vi "Group.Create.vi"(8 "error in (no error)":errorcluster, 9 "Name":string, 11 "Parent":T1 format="%.0x") -> (0 "error out":errorcluster, 2 "Child":T1 format="%.0x", 3 "Parent":T1 format="%.0x")   [LabVIEW 2019, in "Fuel Injector Analysis Addon System Explorer.lvlib"]
uses:
  Fuel Injector Analysis Addon System Explorer.lvlib
  <vilib>/NI VeriStand/Custom Device API/Custom Device Item Ref.ctl
  Addon Shared/Constants.vi
  <vilib>/NI VeriStand/Custom Device Tools/Custom Device Utility Library/NI VeriStand - Search for All Items by GUID.vi
  <vilib>/NI VeriStand/Custom Device Tools/Custom Device Utility Library/Custom Device Utility Library.lvlib
  <vilib>/NI VeriStand/Custom Device API/Custom Device API.lvlib
  Addon Shared/Fuel Injector Analysis Addon Shared.lvlib
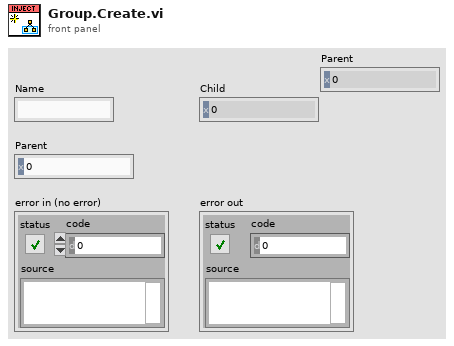
[diagram p1: front panel]
types:
  T1 = typedef "Custom Device API.lvlib/Custom Device Item Ref.ctl" = u64
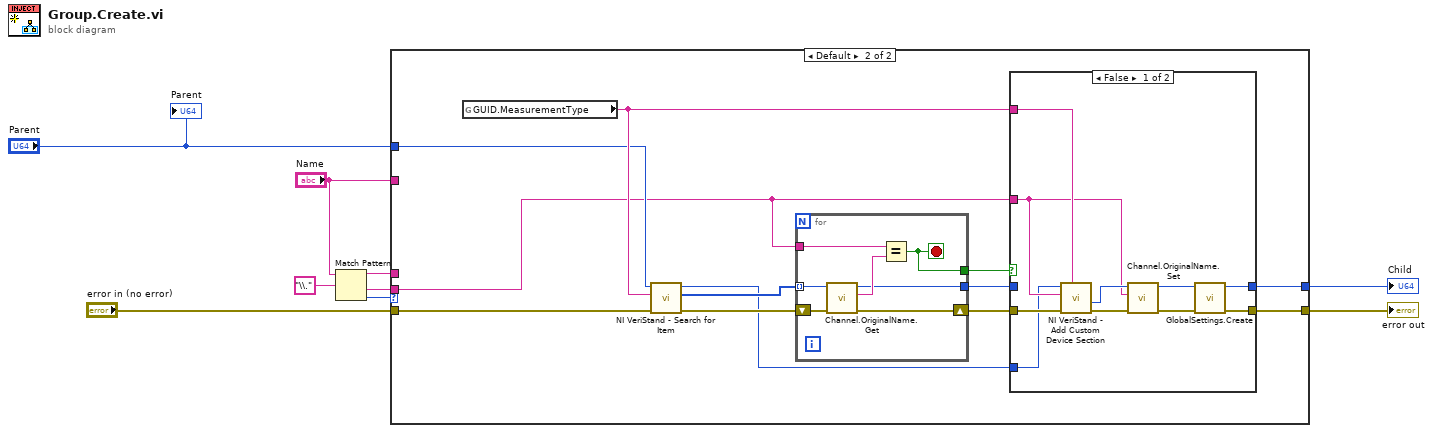
[diagram p0: block diagram]
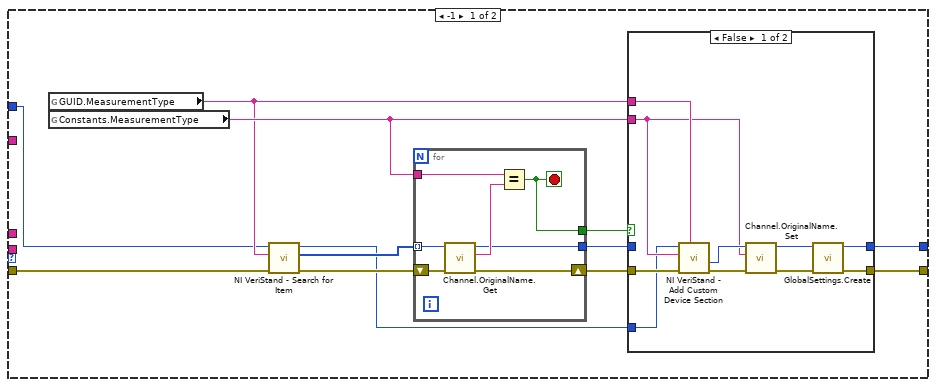
[diagram p2: hidden frame]
diagram:
  n1 = Match Pattern(string="Name", regular expression="\\.") -> (before substring=w4:string, after substring=w9:string, offset past match=w2:i32)  [unwired: 1 in, 1 out]
  n2 = case shown="Default" w2 {
    tunnel: "error in (no error)" -> [w10 w42]
    tunnel: w4 -> [_ _]
    tunnel: "Parent" -> [w11 w43]
    tunnel: [w21 w52] -> w5
    tunnel: [w20 w51] -> w7
    tunnel: "Name" -> [_ _]
    tunnel: w9 -> [_ w41]
    frame -1 {
      n3 = global read "Constants.vi" "GUID.MeasurementType"() -> (w12:string)
      n4 = global read "Constants.vi" "Constants.MeasurementType"() -> (w13:string)
      n5 = call-poly <vilib>:"NI VeriStand - Search for Item.vi"("error in"=w10, "Item GUID"=w12, "Section Ref in"=w11) -> ("error out"=w19:errorcluster, "Item Refs"=w18:T1[], "Section Ref out"=w14:T1)  [unwired: 5 in, 1 out]
      n6 = for {
        shift-right: [w27] -> w17
        shift-left: w19 -> [w28]
        tunnel: w18 -> [w26] mode=indexing
        tunnel: w13 -> [w24]
        tunnel: [w23] -> w15
        tunnel: [w22] -> w16
        stop <- w22 stop-if-true
        n7 = call "Channel.OriginalName.Get.vi"("error in (no error)"=w28, "Ref in"=w26) -> ("error out"=w27:errorcluster, "Value"=w25:string, "Ref out"=w23:T1)  [unwired: 6 in, 1 out]
        n8 = Equal?(x=w24, y=w25) -> (x = y?=w22:bool)
      }
      n9 = case shown="False" w16 {
        tunnel: w17 -> [w38 w40]
        tunnel: w15 -> [_ w39]
        tunnel: [w30 w40] -> w21
        tunnel: [w31 w39] -> w20
        tunnel: w13 -> [w34 _]
        tunnel: w12 -> [w37 _]
        tunnel: w14 -> [w29 _]
        frame False {
          n10 = call <vilib>:"NI VeriStand - Add Custom Device Section.vi"("GUID (Default Section)"=w37, "error in (no error)"=w38, "Section Name"=w34, "Parent Ref in"=w29) -> ("error out"=w35:errorcluster, "Section Ptr"=w36:T1)  [unwired: 4 in, 2 out]
          n11 = call "Channel.OriginalName.Set.vi"("error in (no error)"=w35, "Constants.Channel Name"=w34, "Ref"=w36) -> ("error out"=w33:errorcluster, "Ref out"=w32:T1)  [unwired: 7 in]
          n12 = call "GlobalSettings.Create.vi"("error in (no error)"=w33, "Device Item Ref in"=w32) -> ("error out"=w30:errorcluster, "Parent Ref out"=w31:T1)  [unwired: 8 in]
        }
        frame True {
        }
      }
    }
    frame Default {
      n13 = global read "Constants.vi" "GUID.MeasurementType"() -> (w44:string)
      n14 = call-poly <vilib>:"NI VeriStand - Search for Item.vi"("error in"=w42, "Item GUID"=w44, "Section Ref in"=w43) -> ("error out"=w50:errorcluster, "Item Refs"=w49:T1[], "Section Ref out"=w45:T1)  [unwired: 5 in, 1 out]
      n15 = for {
        shift-right: [w58] -> w48
        shift-left: w50 -> [w59]
        tunnel: w49 -> [w57] mode=indexing
        tunnel: w41 -> [w55]
        tunnel: [w54] -> w46
        tunnel: [w53] -> w47
        stop <- w53 stop-if-true
        n16 = call "Channel.OriginalName.Get.vi"("error in (no error)"=w59, "Ref in"=w57) -> ("error out"=w58:errorcluster, "Value"=w56:string, "Ref out"=w54:T1)  [unwired: 6 in, 1 out]
        n17 = Equal?(x=w55, y=w56) -> (x = y?=w53:bool)
      }
      n18 = case shown="False" w47 {
        tunnel: w48 -> [w69 w71]
        tunnel: w46 -> [_ w70]
        tunnel: [w61 w71] -> w52
        tunnel: [w62 w70] -> w51
        tunnel: w41 -> [w65 _]
        tunnel: w44 -> [w68 _]
        tunnel: w45 -> [w60 _]
        frame False {
          n19 = call <vilib>:"NI VeriStand - Add Custom Device Section.vi"("GUID (Default Section)"=w68, "error in (no error)"=w69, "Section Name"=w65, "Parent Ref in"=w60) -> ("error out"=w66:errorcluster, "Section Ptr"=w67:T1)  [unwired: 4 in, 2 out]
          n20 = call "Channel.OriginalName.Set.vi"("error in (no error)"=w66, "Constants.Channel Name"=w65, "Ref"=w67) -> ("error out"=w64:errorcluster, "Ref out"=w63:T1)  [unwired: 7 in]
          n21 = call "GlobalSettings.Create.vi"("error in (no error)"=w64, "Device Item Ref in"=w63) -> ("error out"=w61:errorcluster, "Parent Ref out"=w62:T1)  [unwired: 8 in]
        }
        frame True {
        }
      }
    }
  }
  "Child" <- w7
  "error out" <- w5
  "Parent" <- "Parent"
